vi "generate_2_c.vi"() -> ()   [LabVIEW 2023]
uses:
  queue_op.ctl
  <vilib>/Utility/error.llb/DialogType.ctl
  global_vars.vi
panel:
  in  "stop":bool
  out "error out 2":errorcluster
  in  "error in":errorcluster
  out "Data":i32
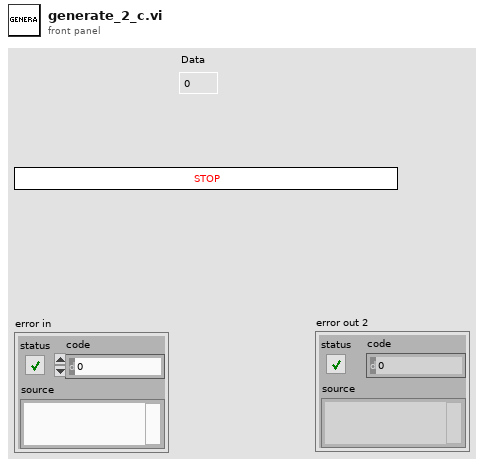
[diagram p1: front panel]
types:
  T1 = typedef "queue_op.ctl" = enum16{"Sum", "Dequeue", "Enqueue", "Initialize"}
  T2 = typedef "DialogType.ctl" = u16
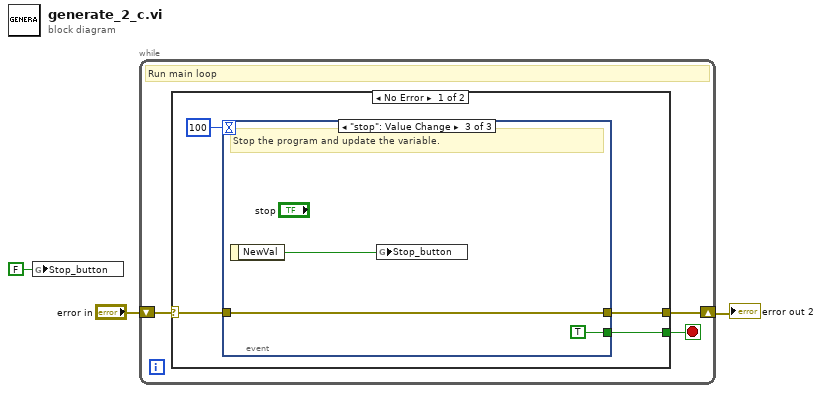
[diagram p0: block diagram]
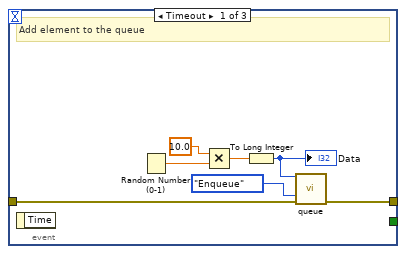
[diagram p2: hidden frame]
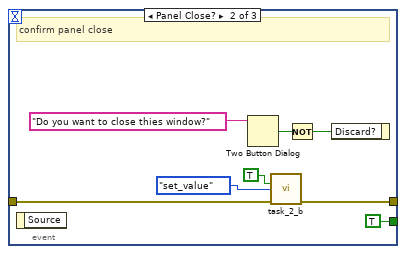
[diagram p3: hidden frame]
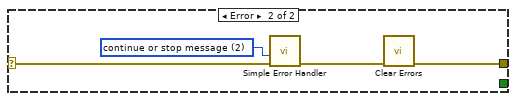
[diagram p4: hidden frame]
diagram:
  n1 = global write "global_vars.vi" "Stop_button"(FALSE ("Stop_button")) -> ()
  n2 = while {
    shift-right: [w5] -> w2
    shift-left: "error in" -> [w6]
    stop <- w4 stop-if-true
    # "Run main loop"
    n3 = case shown="No Error" w6 {
      selector: w6 -> [w9 w32]
      tunnel: [w8 w30] -> w5
      tunnel: [w7 _] -> w4
      frame No Error {
        n4 = event shown="[2] \"stop\": Value Change" {
          selector: _ -> [_ _ _]
          dyn-events: _ -> [_ _ _]
          timeout: 100 -> [_ _ _]
          tunnel: [w13 w21 w28] -> w8
          tunnel: w9 -> [w14 w22 w28]
          tunnel: [_ TRUE TRUE] -> w7
          event Timeout {
            # "Add element to the queue"
            n5 = event-data() -> ()  [unwired: 1 in, 1 out]
            n6 = Random Number (0-1)() -> (number: 0 to 1=w17:dbl)
            n7 = Multiply(x=10.0, y=w17) -> (x*y=w15:dbl)
            n8 = To Long Integer(number=w15) -> (32bit integer=w12:i32)
            "Data" <- w12
            n9 = call "queue.vi"("Input"=w12, "Enum"=queue_op."Enqueue", "error in"=w14) -> ("error out"=w13:errorcluster)  [unwired: 10 in, 2 out]
          }
          event Panel Close? {
            # "confirm panel close"
            n10 = event-data() -> ()  [unwired: 1 in, 1 out]
            n11 = Two Button Dialog(message="Do you want to close thies window?") -> (T button?=w24:bool)  [unwired: 2 in]
            n12 = call "task_2_b.vi"("Stop"=TRUE, "Operation"=enum16{"get_value", "set_value", "Initialize"}."set_value", "error constant"=w22) -> ("error IO"=w21:errorcluster)  [unwired: 10 in, 2 out]
            n13 = Not(x=w24) -> (.not. x?=w23:bool)
            n14 = event-data("Discard?"=w23) -> ()  [unwired: 1 in, 1 out]
          }
          event "stop": Value Change {
            # "Stop the program and update the variable."
            n15 = event-data() -> ("NewVal"=w26:bool)  [unwired: 1 in]
            n16 = global write "global_vars.vi" "Stop_button"(w26) -> ()
          }
        }
      }
      frame Error {
        w29 = T2 2 items=["no dialog", "OK message", "continue or stop message", "OK message + warnings", "continue/stop + warnings"] ("type of dialog (OK msg:1)")
        n17 = call <vilib>:"Simple Error Handler.vi"("type of dialog (OK msg:1)"=w29, "error in (no error)"=w32) -> ("error out"=w31:errorcluster)  [unwired: 3 in, 4 out]
        n18 = call <vilib>:"Clear Errors.vi"("error in (no error)"=w31) -> ("error out"=w30:errorcluster)  [unwired: 5 in, 1 out]
      }
    }
  }
  "error out 2" <- w2
